vi "tlc_Record Dialog Box.vi"(8 "error in (no error)":errorcluster) -> (0 "error out":errorcluster, 2 "Output Cue":T1 {"Channels"."Intensity" min=0.0 max=100.0 step=1.0 format="%#.0f"}, 3 "Cancelled?":bool)   [LabVIEW 2018]
doc: "Use this template to create a dialog box with event handling."
uses:
  Controls/tlc_Cue_Information.ctl
  Controls/channel.ctl
  Modules/Cue/tlc_Cue_Information Command.ctl
panel:
  in  "Cue Information":T1 {"Channels"."Intensity" min=0.0 max=100.0 step=1.0 format="%#.0f"}
  in  "Cancel":bool
  in  "OK":bool
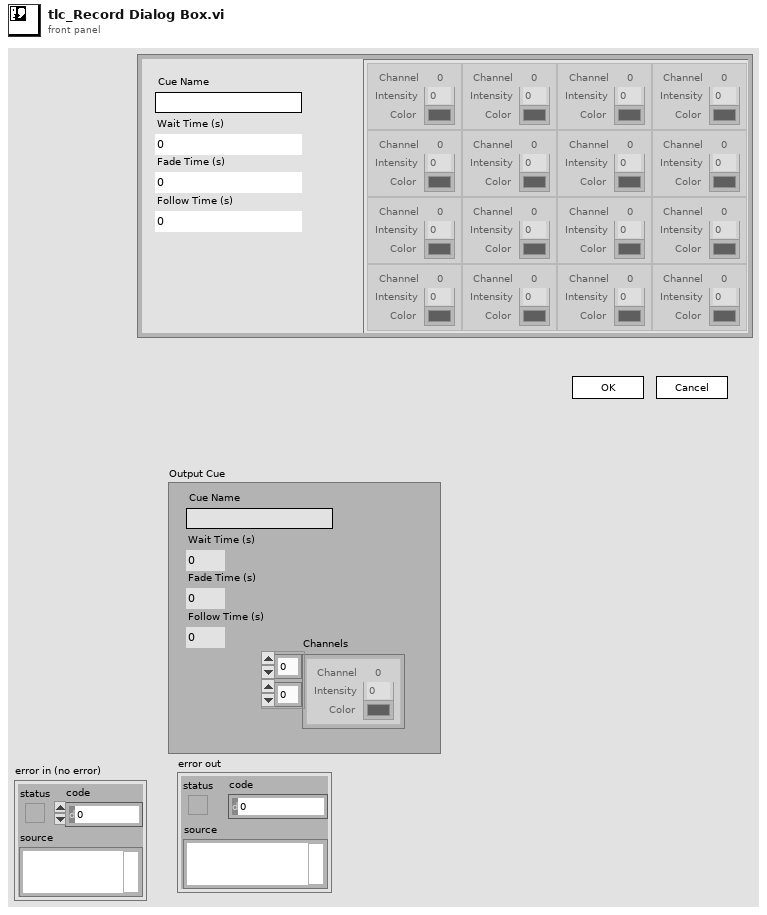
[diagram p1: front panel]
types:
  T1 = typedef "tlc_Cue_Information.ctl" = cluster{"Cue Name":string, "Wait Time (s)":u32, "Fade Time (s)":u32, "Follow Time (s)":u32, "Channels":T2[][]}
  T2 = typedef "channel.ctl" = cluster{"Intensity":dbl, " Color":u32, "Channel":i32}
  T3 = typedef "tlc_Cue_Information Command.ctl" = enum16{"Add Cue", "Delete Cue", "Get Cue Values", "Set Cue Values", "Swap", "Get Number of Cues", "Initialize", "Get Empty Cue"}
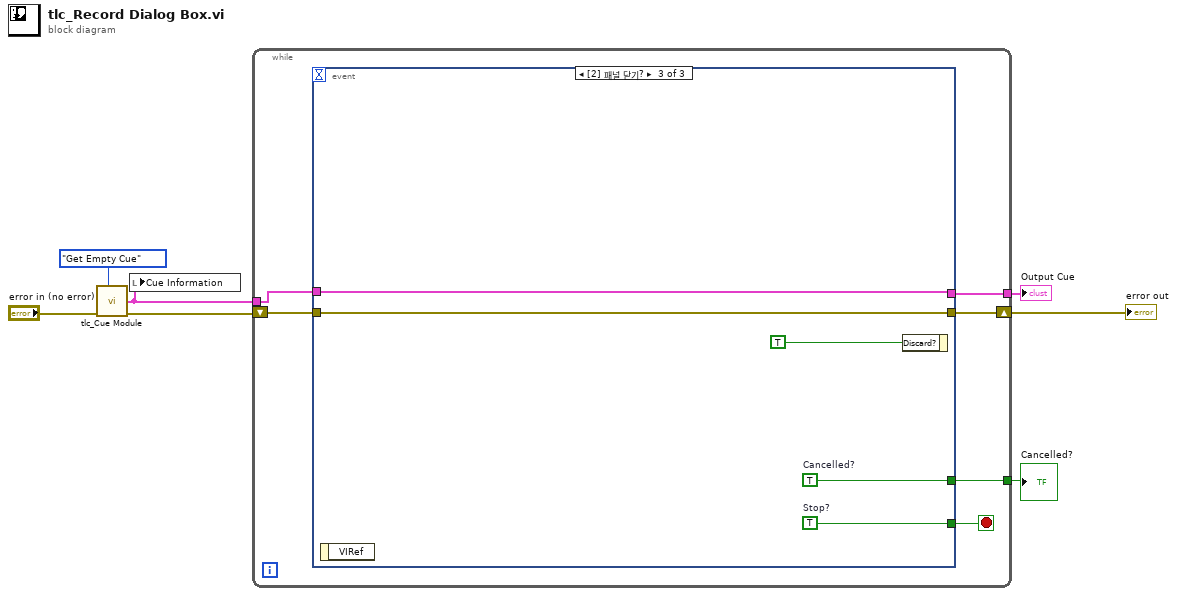
[diagram p0: block diagram]
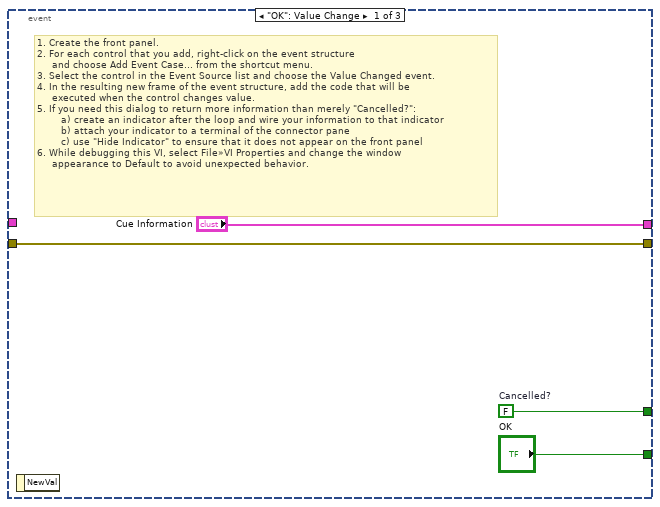
[diagram p2: hidden frame]
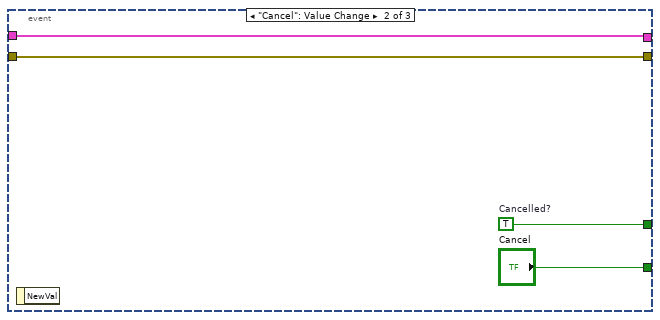
[diagram p3: hidden frame]
diagram:
  n1 = call "tlc_Cue Module.vi"("Command"=tlc_Cue_Information_Command."Get Empty Cue", "error in (no error)"="error in (no error)") -> ("error out"=w6:errorcluster, "Cue Output"=w4:T1)  [unwired: 6 in, 1 out]
  n2 = local write "Cue Information"(w4) -> ()
  n3 = while {
    tunnel: [w12] -> w7
    tunnel: [w11] -> w1
    shift-right: [w9] -> w2
    shift-left: w6 -> [w8]
    tunnel: w4 -> [w10]
    stop <- w13 stop-if-true
    n4 = event shown="[2] 패널 닫기?" {
      selector: _ -> [_ _ _]
      dyn-events: _ -> [_ _ _]
      timeout: _ -> [_ _ _]
      tunnel: ["OK" "Cancel" w25] -> w13
      tunnel: [w17 w21 w24] -> w12
      tunnel: ["Cue Information" w19 w23] -> w11
      tunnel: w10 -> [_ w19 w23]
      tunnel: [w14 w18 w22] -> w9
      tunnel: w8 -> [w14 w18 w22]
      event "OK": Value Change {
        w17 = FALSE  # Cancelled?
        # "1. Create the front panel.\n2. For each control that you add, right-click on the event structure \n     and choose Add Event Case... from the shortcut menu.\n3. Select the control in the Event Source list and choose the Value Changed event.\n4. In the resulting new frame of the event structure, add the code that will be \n     executed when the control changes value.\n5. If you need this dialog to return more information than merely \"Cancelled?\":\n        a) create an indicator after the loop and wire your information to that indicator\n        b) attach your indicator to a terminal of the connector pane\n        c) use \"Hide Indicator\" to ensure that it does not appear on the front panel\n6. While debugging this VI, select File»VI Properties and change the window \n     appearance to Default to avoid unexpected behavior."
        n5 = event-data() -> ()  [unwired: 1 in, 1 out]
      }
      event "Cancel": Value Change {
        w21 = TRUE  # Cancelled?
        n6 = event-data() -> ()  [unwired: 1 in, 1 out]
      }
      event Panel Close? {
        w24 = TRUE  # Cancelled?
        w25 = TRUE  # Stop?
        n7 = event-data() -> ()  [unwired: 1 in, 1 out]
        n8 = event-data("Discard?"=TRUE) -> ()  [unwired: 1 in, 1 out]
      }
    }
  }
  "Cancelled?" <- w7
  "error out" <- w2
  "Output Cue" <- w1
